vi "Update Steering Motor Angle State.vi"(8 "error in (no error)":errorcluster, 10 "ccw motor angle state (rad)":dbl, 11 "wheel in":refnum<class "NI_Robotics_Wheel.lvclass">) -> (0 "error out":errorcluster, 1 "failed?":bool, 3 "wheel out":refnum<class "NI_Robotics_Wheel.lvclass">)   [LabVIEW 2017, in "NI_Robotics_Wheel.lvclass"]
uses:
  <vilib>/robotics/Steering/Wheel/NI_Robotics_Wheel.lvclass
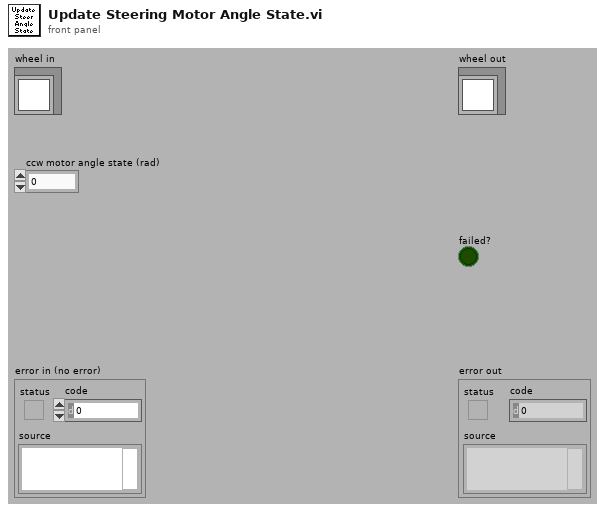
[diagram p1: front panel]
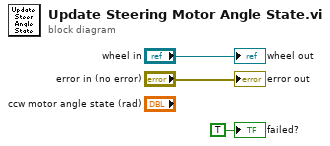
[diagram p0: block diagram]
diagram:
  "error out" <- "error in (no error)"
  "wheel out" <- "wheel in"
  "failed?" <- TRUE ("failed?")
